vi "Receive String Value Msg.vi"(8 "error in (no error)":errorcluster, 10 "StringValueMsg":refnum<class "StringValueMsg.lvclass">, 11 "TopLevelApplication in":refnum<class "TopLevelApplication.lvclass">) -> (0 "error out":errorcluster, 3 "TopLevelApplication out":refnum<class "TopLevelApplication.lvclass">)   [LabVIEW 2015, in "TopLevelApplication.lvlib" / "TopLevelApplication.lvclass"]
uses:
  TopLevelApplication.lvclass
  AutoRegistration/ActorAutoRegistration Messages/StringValueMsg/StringValueMsg.lvclass
  Dialog Box Implementations/OneButtonDialogBox/OneButtonDialogBox.lvclass
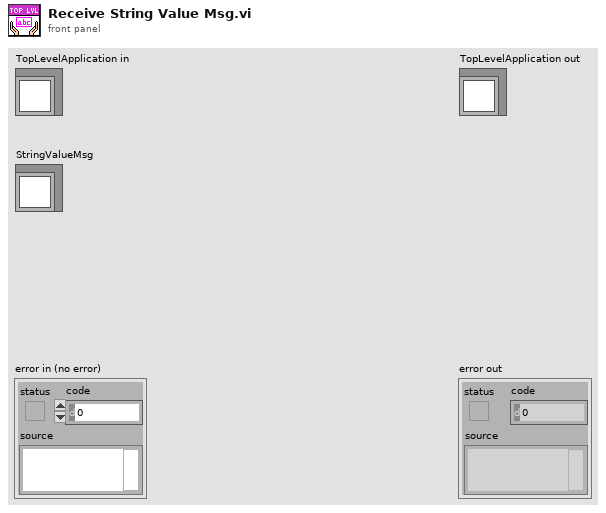
[diagram p1: front panel]
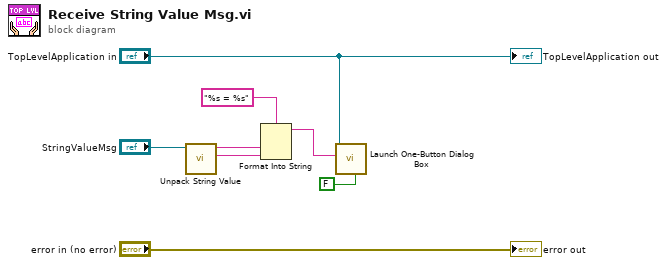
[diagram p0: block diagram]
diagram:
  n1 = call-dynamic "Unpack String Value.vi"("StringValueMsg in"="StringValueMsg") -> ("Value"=w3:string, "Name"=w4:string)  [unwired: 9 in]
  n2 = Format Into String(format string="%s = %s", w4, w3) -> (resulting string=w5:string)  [unwired: 2 in, 1 out]
  n3 = call "Launch One-Button Dialog Box.vi"("Modal? (T)"=FALSE, "Message Text"=w5, "Dialog Launcher"="TopLevelApplication in") -> ()  [unwired: 8 in, 1 out]
  "error out" <- "error in (no error)"
  "TopLevelApplication out" <- "TopLevelApplication in"
